vi "Map_interpolateXYZ.vi"(3 "Level":i32=1, 4 "MapData (2D)":dbl[][](array[numeric]), 5 "XY Unique":cluster{"X Unique":dbl[], "Y Unique":dbl[]}) -> (0 "Z Interpoliert":dbl[][](array[numeric]), 1 "Axes":T1, 2 "XY Unique Interpoliert":cluster{"X Unique":dbl[], "Y Unique":dbl[]})   [LabVIEW 2010]
uses:
  <vilib>/gmath/interp.llb/Interpolate 2D (1d X,Y).vi
  <vilib>/gmath/NI_Gmath.lvlib
panel:
  out "Fehler":errorcluster caption="Fehler (Ausgang)"
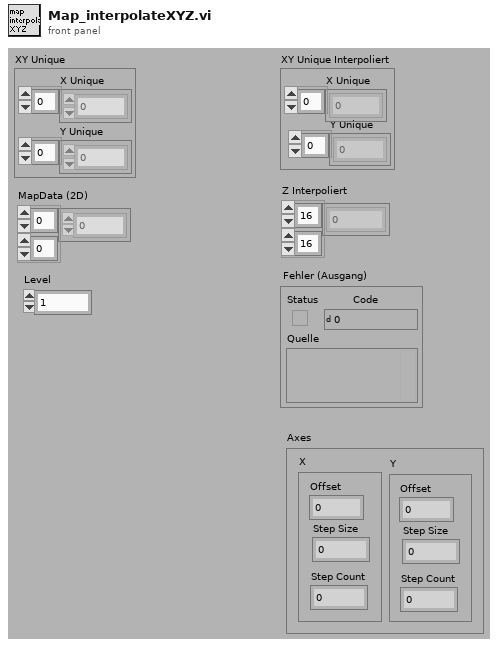
[diagram p1: front panel]
types:
  T1 = cluster{"X":cluster{"Offset":dbl, "Step Size":dbl, "Step Count":i32}, "Y":cluster{"Offset":dbl, "Step Size":dbl, "Step Count":i32}}
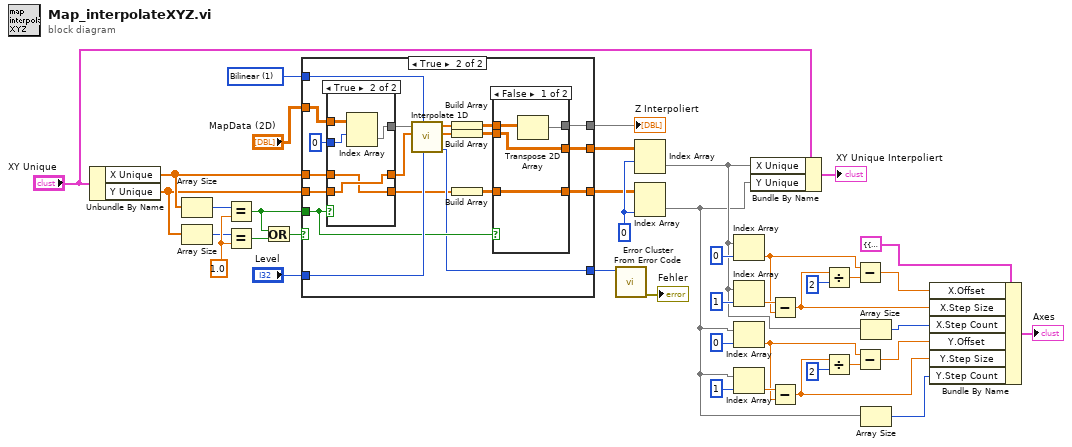
[diagram p0: block diagram]
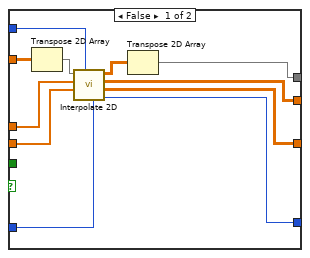
[diagram p2: hidden frame]
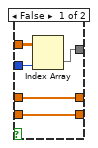
[diagram p4: hidden frame]
diagram:
  w37 = 1.0 ("y")
  w41 = 0 ("Index")
  w31 = 1 items=["Nächste", "Bilinear", "Bikubisch", "Spline (bikubisch)"] ("method")
  n1 = Unbundle By Name("XY Unique") -> ("X Unique"=w29:dbl[], "Y Unique"=w28:dbl[])
  n2 = Array Size(array=w29) -> (size(s)=w36:i32)
  n3 = Array Size(array=w28) -> (size(s)=w35:i32)
  n4 = Equal?(x=w36, y=w37) -> (x = y?=w33:bool)
  n5 = Equal?(x=w35, y=w37) -> (x = y?=w38:bool)
  n6 = Or(x=w33, y=w38) -> (x .or. y?=w34:bool)
  n7 = case shown="True" w34 {
    tunnel: w33 -> [_ w67]
    tunnel: "Level" -> [w52 w71]
    tunnel: w31 -> [w51 w70]
    tunnel: "MapData (2D)" -> [w45 w57]
    tunnel: w29 -> [w50 w63]
    tunnel: w28 -> [w49 w69]
    tunnel: [w42 w64] -> w27
    tunnel: [w48 w62] -> w24
    tunnel: [w47 w54] -> w26
    tunnel: [w46 w53] -> w25
    frame False {
      n8 = Transpose 2D Array(2D array=w45) -> (transposed array=w44:dbl[][])
      n9 = call-poly <vilib>:"Interpolate 2D.vi"("ntimes"=w52, "method"=w51, "Y"=w49, "X"=w50, "Z"=w44) -> ("error"=w48:i32, "yi used"=w46:dbl[][], "xi used"=w47:dbl[][], "zi"=w43:dbl[][])  [unwired: 3 in]
      n10 = Transpose 2D Array(2D array=w43) -> (transposed array=w42:dbl[][])
    }
    frame True {
      n11 = case shown="True" w67 {
        tunnel: [w83 w88] -> w68
        tunnel: w63 -> [w83 w87]
        tunnel: w69 -> [w82 w88]
        tunnel: [w82 w87] -> w60
        tunnel: [w80 w86] -> w55
        tunnel: w57 -> [w81 w85]
        tunnel: 0 ("Index") -> [w79 w84]
        frame False {
          n12 = Index Array(array=w81, index (col)=w79) -> (element=w80:dbl[])  [unwired: 1 in]
        }
        frame True {
          n13 = Index Array(array=w85, index (row)=w84) -> (element=w86:dbl[])  [unwired: 1 in]
        }
      }
      n14 = call <vilib>:"Interpolate 1D.vi"("ntimes"=w71, "method"=w70, "X"=w68, "Y"=w55) -> ("error"=w62:i32, "xi used"=w59:dbl[], "yi"=w66:dbl[])  [unwired: 5 in]
      n15 = Build Array(w66) -> (w65:dbl[][])
      n16 = Build Array(w59) -> (w58:dbl[][])
      n17 = Build Array(w60) -> (w61:dbl[][])
      n18 = case shown="False" w67 {
        tunnel: w65 -> [w73 w76]
        tunnel: [w72 w76] -> w64
        tunnel: w58 -> [w75 w78]
        tunnel: [w74 w78] -> w53
        tunnel: [w75 w77] -> w54
        tunnel: w61 -> [w74 w77]
        frame False {
          n19 = Transpose 2D Array(2D array=w73) -> (transposed array=w72:dbl[][])
        }
        frame True {
        }
      }
    }
  }
  "Z Interpoliert" <- w27
  n20 = call <vilib>:"Error Cluster From Error Code.vi"("error code (0)"=w24) -> ("error out"=→"Fehler":errorcluster)  [unwired: 8 in]
  n21 = Index Array(array=w26, index (row)=w41) -> (element=w4:dbl[])  [unwired: 1 in]
  n22 = Index Array(array=w25, index (col)=w41) -> (element=w3:dbl[])  [unwired: 1 in]
  n23 = Index Array(array=w4, index=0) -> (element=w9:dbl)
  n24 = Index Array(array=w4, index=1) -> (element=w18:dbl)
  n25 = Index Array(array=w3, index=0) -> (element=w8:dbl)
  n26 = Index Array(array=w3, index=1) -> (element=w17:dbl)
  n27 = Bundle By Name(cluster="XY Unique", "X Unique"=w4, "Y Unique"=w3) -> (→"XY Unique Interpoliert":cluster{"X Unique":dbl[], "Y Unique":dbl[]})
  n28 = Subtract(x=w18, y=w9) -> (x-y=w10:dbl)
  n29 = Subtract(x=w17, y=w8) -> (x-y=w5:dbl)
  n30 = Divide(x=w10, y=i8 2) -> (x/y=w14:dbl)
  n31 = Divide(x=w5, y=i8 2) -> (x/y=w7:dbl)
  n32 = Subtract(x=w9, y=w14) -> (x-y=w12:dbl)
  n33 = Subtract(x=w8, y=w7) -> (x-y=w13:dbl)
  n34 = Array Size(array=w4) -> (size(s)=w2:i32)
  n35 = Array Size(array=w3) -> (size(s)=w1:i32)
  n36 = Bundle By Name(cluster=T1 {"X"={"Offset"=0.0, "Step Size"=0.0, "Step Count"=0}, "Y"={"Offset"=0.0, "Step Size"=0.0, "Step Count"=0}} ("Axes"), "X.Offset"=w12, "X.Step Size"=w10, "X.Step Count"=w2, "Y.Offset"=w13, "Y.Step Size"=w5, "Y.Step Count"=w1) -> (→"Axes":T1)
